vi "Store Spectrometer ID.vi"(0 "VISA resource name":refnum<visa-resource-name>, 5 "Pixel Mode (0:Optical)":u16(ring) items=["Optical ", "All Pixels"], 9 "Check Vrn First Call (False)":bool, 11 "error in (no error)":errorcluster) -> (4 "VISA resource name out":refnum<visa-resource-name>, 6 "USB Speed":u16, 8 "ID":u16, 10 "Optical Pixels":bool, 15 "error out":errorcluster)   [LabVIEW 2019, in "Ocean Optics 2000 4000.lvlib"]
doc: "Saves the Spectrometer ID and also stores the visa resource name. These are used to look up the ID and pixels (all or optical)."
uses:
  Ocean Optics 2000 4000.lvlib
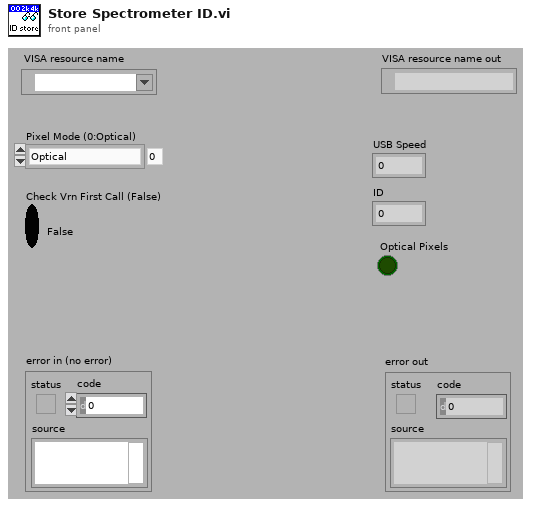
[diagram p1: front panel]
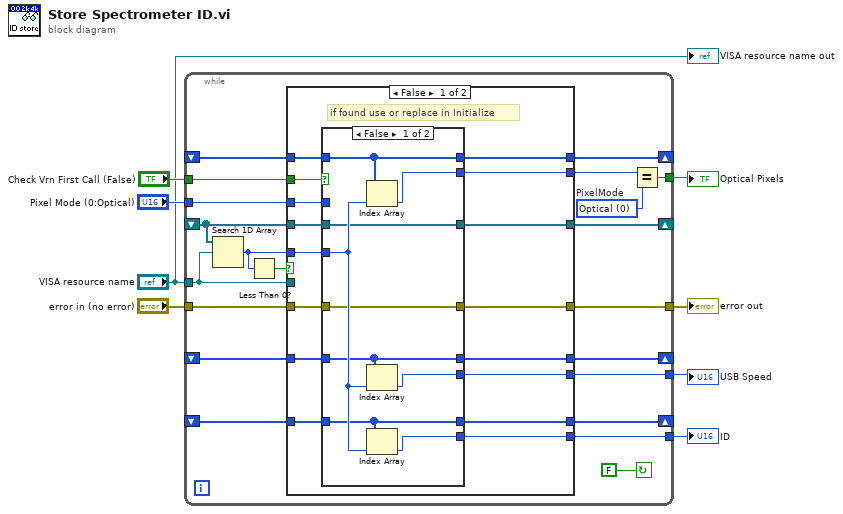
[diagram p0: block diagram]
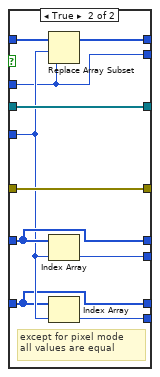
[diagram p2: hidden frame]
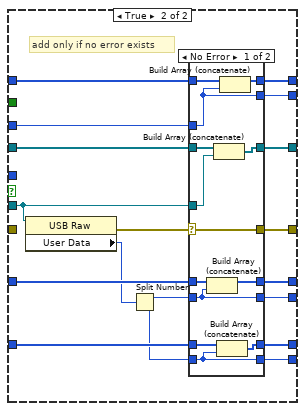
[diagram p3: hidden frame]
diagram:
  n1 = while {
    tunnel: "Pixel Mode (0:Optical)" -> [w28]
    tunnel: "VISA resource name" -> [w26]
    shift-right: [w24] -> _
    shift-left: _ -> [w29]
    shift-right: [w23] -> _
    shift-left: _ -> [w27]
    shift-right: [w22] -> _
    shift-left: _ -> [w21]
    tunnel: [w20] -> w6
    tunnel: "error in (no error)" -> [w19]
    tunnel: [w15] -> w5
    shift-right: [w13] -> _
    shift-left: _ -> [w14]
    tunnel: [w12] -> w4
    tunnel: [w11] -> w3
    tunnel: "Check Vrn First Call (False)" -> [w9]
    stop <- FALSE continue-if-true
    w17 = u16 0 items=["Optical ", "All Pixels"]  # PixelMode
    n2 = Search 1D Array(1D array=w27, element=w26) -> (index of element=w10:i32)  [unwired: 1 in]
    n3 = Less Than 0?(x=w10) -> (x < 0?=w25:bool)
    n4 = case shown="False" w25 {
      tunnel: w29 -> [w44 w82]
      tunnel: [w35 w81] -> w24
      tunnel: [w36 w80] -> w23
      tunnel: w28 -> [w30 w74]
      tunnel: w27 -> [w38 w75]
      tunnel: w26 -> [_ w76]
      tunnel: [w34 w79] -> w22
      tunnel: w21 -> [w43 w78]
      tunnel: [w32 w69] -> w20
      tunnel: w19 -> [w37 _]
      tunnel: [w45 w65] -> w16
      tunnel: w14 -> [w41 w73]
      tunnel: [w31 w72] -> w13
      tunnel: [w40 w66] -> w12
      tunnel: [w42 w67] -> w11
      tunnel: w10 -> [w39 _]
      tunnel: w9 -> [w33 _]
      frame False {
        # "if found use or replace in Initialize"
        n5 = case shown="False" w33 {
          tunnel: [w54 w55] -> w45
          tunnel: w44 -> [w50 w63]
          tunnel: w43 -> [w47 w59]
          tunnel: [w53 w62] -> w42
          tunnel: w41 -> [w46 w57]
          tunnel: [w52 w61] -> w40
          tunnel: w39 -> [w51 w58]
          tunnel: [w50 w56] -> w35
          tunnel: w38 -> [w49 w60]
          tunnel: [w49 w60] -> w36
          tunnel: w37 -> [w48 w64]
          tunnel: [w48 w64] -> w32
          tunnel: [w47 w59] -> w34
          tunnel: [w46 w57] -> w31
          tunnel: w30 -> [_ w55]
          frame False {
            n6 = Index Array(array=w50, index=w51) -> (element=w54:u16)
            n7 = Index Array(array=w47, index=w51) -> (element=w53:u16)
            n8 = Index Array(array=w46, index=w51) -> (element=w52:u16)
          }
          frame True {
            # "except for pixel mode\nall values are equal"
            n9 = Replace Array Subset(array=w63, new element=w55, index=w58) -> (w56:u16[])
            n10 = Index Array(array=w59, index=w58) -> (element=w62:u16)
            n11 = Index Array(array=w57, index=w58) -> (element=w61:u16)
          }
        }
      }
      frame True {
        # "add only if no error exists"
        n12 = property class="USB Raw"(reference=w76) -> (error out=w70:errorcluster, "User Data"=w77:u32)  [unwired: 1 in, 1 out]
        n13 = Split Number(x=w77) -> (hi(x)=w68:u16, lo(x)=w71:u16)
        n14 = case shown="No Error" w70 {
          selector: w70 -> [w86 w101]
          tunnel: w82 -> [w95 w103]
          tunnel: [w94 w103] -> w81
          tunnel: [w93 w102] -> w80
          tunnel: [w92 w100] -> w79
          tunnel: w78 -> [w91 w100]
          tunnel: w76 -> [w90 _]
          tunnel: w75 -> [w89 w102]
          tunnel: w74 -> [w83 w96]
          tunnel: w73 -> [w88 w99]
          tunnel: [w87 w99] -> w72
          tunnel: w71 -> [w84 w98]
          tunnel: w68 -> [w85 w97]
          tunnel: [w86 w101] -> w69
          tunnel: [w85 w97] -> w67
          tunnel: [w84 w98] -> w66
          tunnel: [w83 w96] -> w65
          frame No Error {
            n15 = Build Array (concatenate)(w91, w85) -> (w92:u16[])
            n16 = Build Array (concatenate)(w89, w90) -> (w93:refnum<visa-resource-name>[])
            n17 = Build Array (concatenate)(w88, w84) -> (w87:u16[])
            n18 = Build Array (concatenate)(w95, w83) -> (w94:u16[])
          }
          frame Error {
          }
        }
      }
    }
    n19 = Equal?(x=w16, y=w17) -> (x = y?=w15:bool)
  }
  "error out" <- w6
  "Optical Pixels" <- w5
  "ID" <- w4
  "USB Speed" <- w3
  "VISA resource name out" <- "VISA resource name"
